vi "基本参数计算.vi"(10 "temp实际摄氏温度":dbl, 11 "atm/kPa":dbl) -> (2 "实际空气密度":dbl, 3 "Z0空气的特性阻抗":dbl, 5 "考虑温度实际声速c0":dbl)   [LabVIEW 2018]
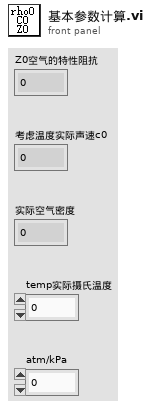
[diagram p1: front panel]
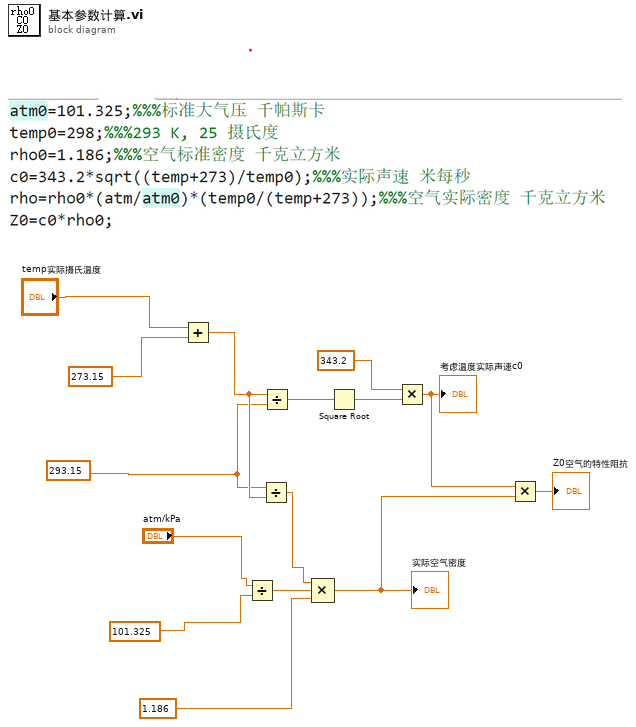
[diagram p0: block diagram]
diagram:
  w3 = 293.15 ("y")
  n1 = Add(x="temp实际摄氏温度", y=273.15) -> (x+y=w8:dbl)
  n2 = Divide(x="atm/kPa", y=101.325) -> (x/y=w9:dbl)
  n3 = Divide(x=w3, y=w8) -> (x/y=w7:dbl)
  n4 = Divide(x=w8, y=w3) -> (x/y=w13:dbl)
  n5 = Compound Arithmetic op=MULTIPLY(w7, w9, 1.186 ("值")) -> (w5:dbl)
  "实际空气密度" <- w5
  n6 = Square Root(x=w13) -> (sqrt(x)=w12:dbl)
  n7 = Multiply(x=343.2, y=w12) -> (x*y=w6:dbl)
  "考虑温度实际声速c0" <- w6
  n8 = Multiply(x=w6, y=w5) -> (x*y=→"Z0空气的特性阻抗":dbl)
